vi "GetParameterNames.vi"(8 "error in (no error)":errorcluster, 11 "Aerotech_Soloist in":refnum<class "Aerotech_Soloist.lvclass">) -> (0 "error out":errorcluster, 2 "Parameter Set Name":string[](array[string]), 3 "Aerotech_Soloist out":refnum<class "Aerotech_Soloist.lvclass">)   [LabVIEW 2013, in "Aerotech_Soloist.lvclass"]
uses:
  Aerotech_Soloist.lvclass
  Aerotech_Soloist.lvclass/Aerotech_Soloist.ctl
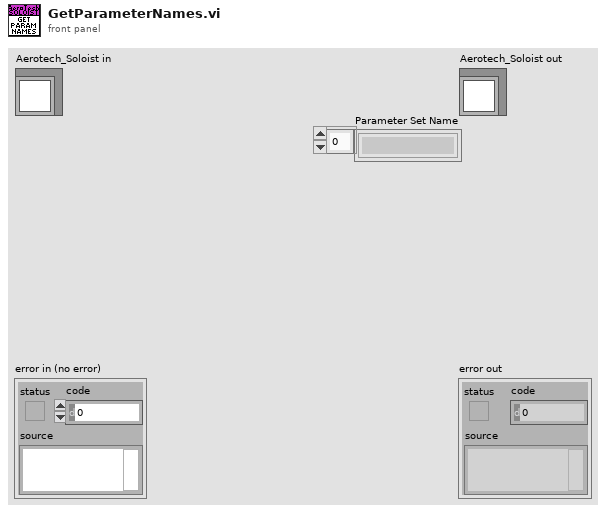
[diagram p1: front panel]
types:
  T1 = typedef "Aerotech_Soloist.lvclass/ParameterSet.ctl" = cluster{"Name":string, "SCurve %":dbl, "Ramp Mode":string, "Ramp Value":dbl}
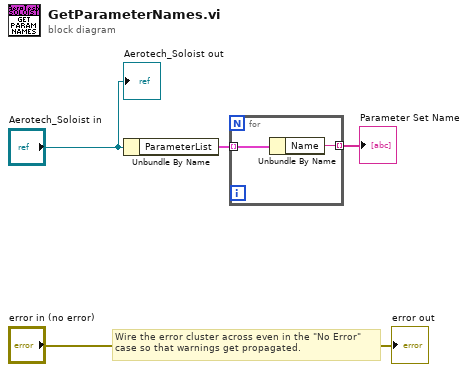
[diagram p0: block diagram]
diagram:
  # "Wire the error cluster across even in the \"No Error\"\ncase so that warnings get propagated."
  n1 = Unbundle By Name("Aerotech_Soloist in") -> ("ParameterList"=w2:T1[])
  n2 = for {
    tunnel: w2 -> [w6] mode=indexing
    tunnel: [w5] -> w1 mode=indexing
    n3 = Unbundle By Name(w6) -> ("Name"=w5:string)
  }
  "Parameter Set Name" <- w1
  "error out" <- "error in (no error)"
  "Aerotech_Soloist out" <- "Aerotech_Soloist in"
